vi "CreateExperimentRunTotalChargeNode.vi"(8 "Error In":errorcluster, 10 "Experiment Run Total Charge (C)":T1={"Start"=nan, "Stop"=nan}, 11 "DOM Document In":refnum<k20>) -> (0 "Error out":errorcluster, 2 "Experiment Run Total Charge Node":refnum<k20>, 3 "DOM Document Out":refnum<k20>)   [LabVIEW 2012]
uses:
  ExperimentRunTotalCharge.ctl
  <resource>/objmgr/DOMUserDefRef.rc
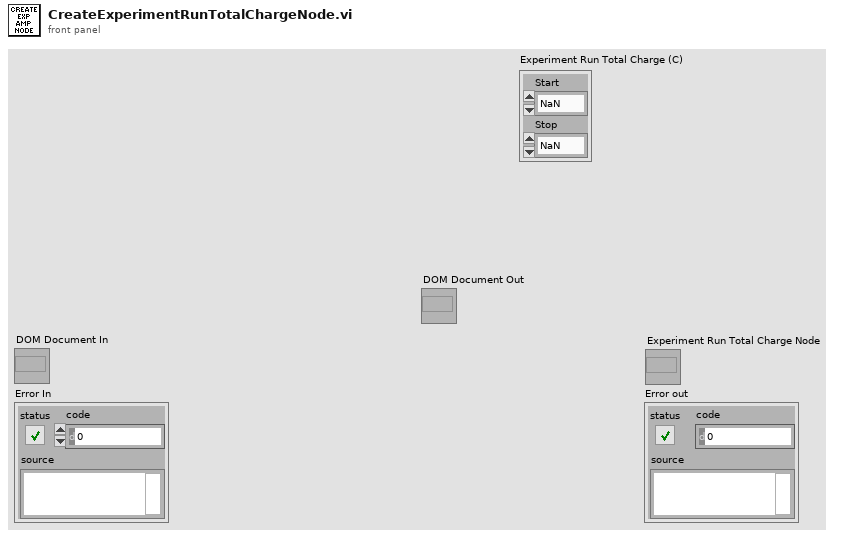
[diagram p1: front panel]
types:
  T1 = typedef "ExperimentRunTotalCharge.ctl" = cluster{"Start":dbl, "Stop":dbl}
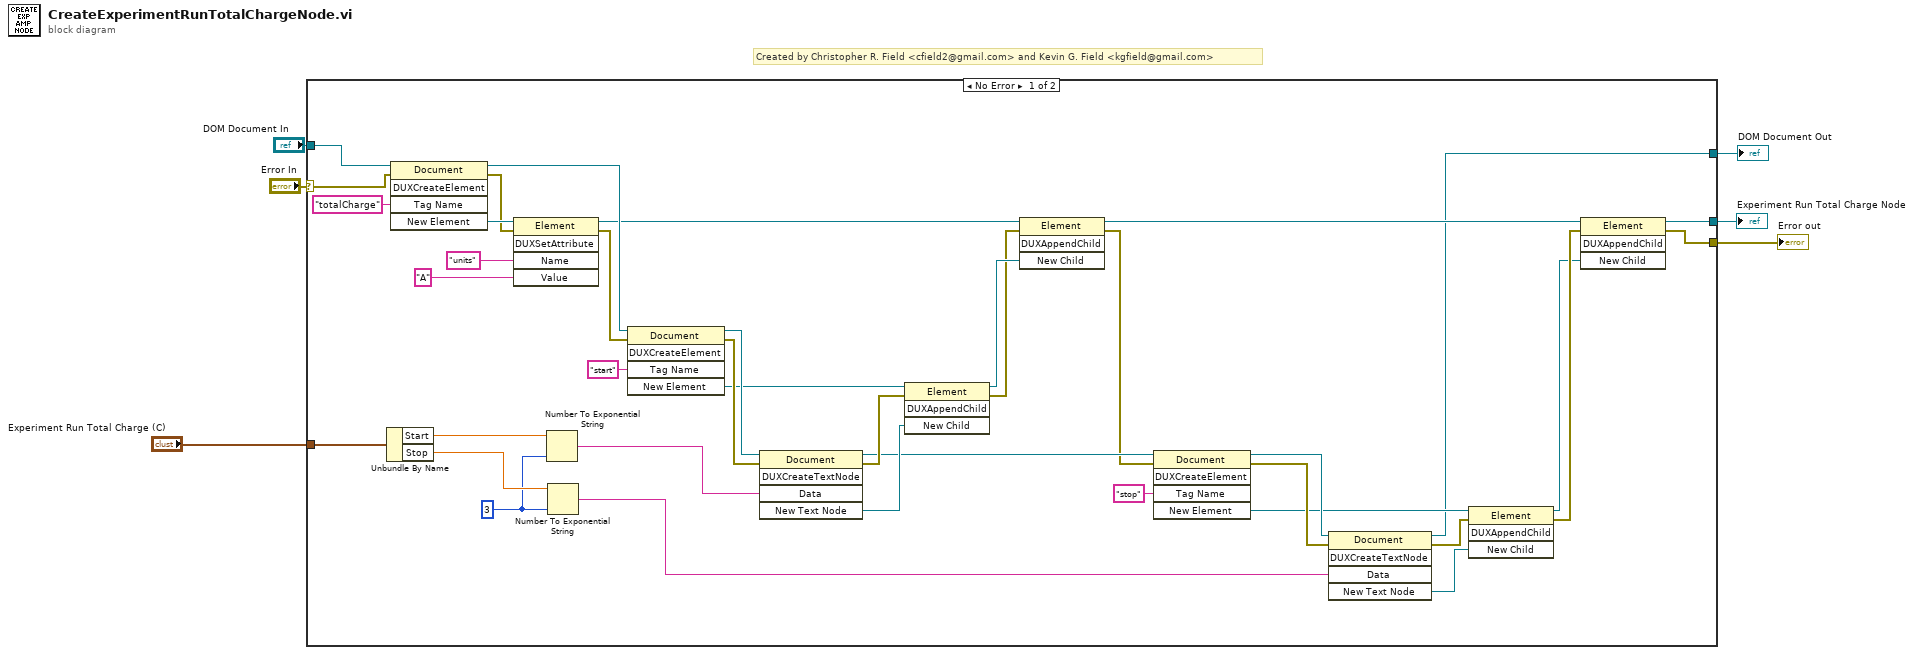
[diagram p0: block diagram]
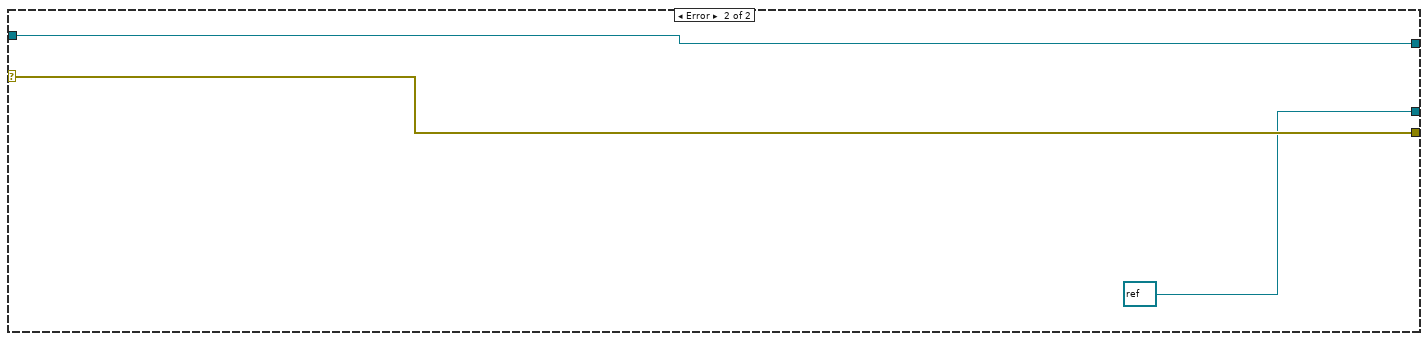
[diagram p2: hidden frame]
diagram:
  # "Created by Christopher R. Field <cfield2@gmail.com> and Kevin G. Field <kgfield@gmail.com>"
  n1 = case shown="No Error" "Error In" {
    selector: "Error In" -> [w41 w46]
    tunnel: "DOM Document In" -> [w44 w47]
    tunnel: [w21 refnum<k20> refnum ("Operator Node 2")] -> w5
    tunnel: [w19 w46] -> w4
    tunnel: [w20 w47] -> w2
    tunnel: "Experiment Run Total Charge (C)" -> [w40 _]
    frame No Error {
      w9 = i16 3 ("precision (6)")
      n2 = Unbundle By Name(w40) -> ("Start"=w11:dbl, "Stop"=w10:dbl)
      n3 = invoke class="Document" method="DUXCreateElement"(reference=w44, error in=w41, "Tag Name"="totalCharge") -> (reference out=w14:refnum<k20>, error out=w15:errorcluster, "New Element"=w18:refnum<k20>)  [unwired: 2 in, 2 out]
      n4 = invoke class="Element" method="DUXSetAttribute"(reference=w18, error in=w15, "Name"="units", "Value"="A" ("Attribute Value")) -> (reference out=w12:refnum<k20>, error out=w13:errorcluster)  [unwired: 1 in, 3 out]
      n5 = Number To Exponential String(number=w11, precision (6)=w9) -> (E-format string=w8:string)  [unwired: 2 in]
      n6 = Number To Exponential String(number=w10, precision (6)=w9) -> (E-format string=w7:string)  [unwired: 2 in]
      n7 = invoke class="Document" method="DUXCreateElement"(reference=w14, error in=w13, "Tag Name"="start") -> (reference out=w38:refnum<k20>, error out=w37:errorcluster, "New Element"=w36:refnum<k20>)  [unwired: 2 in, 2 out]
      n8 = invoke class="Document" method="DUXCreateTextNode"(reference=w38, error in=w37, "Data"=w8) -> (reference out=w32:refnum<k20>, error out=w35:errorcluster, "New Text Node"=w42:refnum<k20>)  [unwired: 2 in, 2 out]
      n9 = invoke class="Element" method="DUXAppendChild"(reference=w36, error in=w35, "New Child"=w42) -> (reference out=w34:refnum<k20>, error out=w33:errorcluster)  [unwired: 1 in, 2 out]
      n10 = invoke class="Element" method="DUXAppendChild"(reference=w12, error in=w33, "New Child"=w34) -> (reference out=w22:refnum<k20>, error out=w31:errorcluster)  [unwired: 1 in, 2 out]
      n11 = invoke class="Document" method="DUXCreateElement"(reference=w32, error in=w31, "Tag Name"="stop") -> (reference out=w29:refnum<k20>, error out=w28:errorcluster, "New Element"=w27:refnum<k20>)  [unwired: 2 in, 2 out]
      n12 = invoke class="Document" method="DUXCreateTextNode"(reference=w29, error in=w28, "Data"=w7) -> (reference out=w20:refnum<k20>, error out=w26:errorcluster, "New Text Node"=w25:refnum<k20>)  [unwired: 2 in, 2 out]
      n13 = invoke class="Element" method="DUXAppendChild"(reference=w27, error in=w26, "New Child"=w25) -> (reference out=w23:refnum<k20>, error out=w24:errorcluster)  [unwired: 1 in, 2 out]
      n14 = invoke class="Element" method="DUXAppendChild"(reference=w22, error in=w24, "New Child"=w23) -> (reference out=w21:refnum<k20>, error out=w19:errorcluster)  [unwired: 1 in, 2 out]
    }
    frame Error {
    }
  }
  "Experiment Run Total Charge Node" <- w5
  "Error out" <- w4
  "DOM Document Out" <- w2
